vi "Keithley 2600 Series Current Sweep Script.vi"() -> ()   [LabVIEW 2020]
doc: "This example shows how to create, run a script and query the script output data."
uses:
  Keithley 2600 Series.lvlib
panel:
  out "Array":string[](array[string])
  out "error out":errorcluster
  out "Last Measured Voltage (V)":dbl
  out "Voltage Measurements (V)":string
  in  "Source Code":string="smua.reset()\nsmua.source.limitv = 1\nSweepILinMeasureV(smua, 0.01, 0.1, 0.2, 10)\nprintbuffer(1, 10, smua.nvbuffer1)\nprint(smua.nvbuffer1.readings[10])\n"
  in  "Script Variable (myScript)":string="myScript"
  in  "VISA resource name":refnum<visa-resource-name>
  # "(c) 2020 National Instruments.  ALL RIGHTS RESERVED."
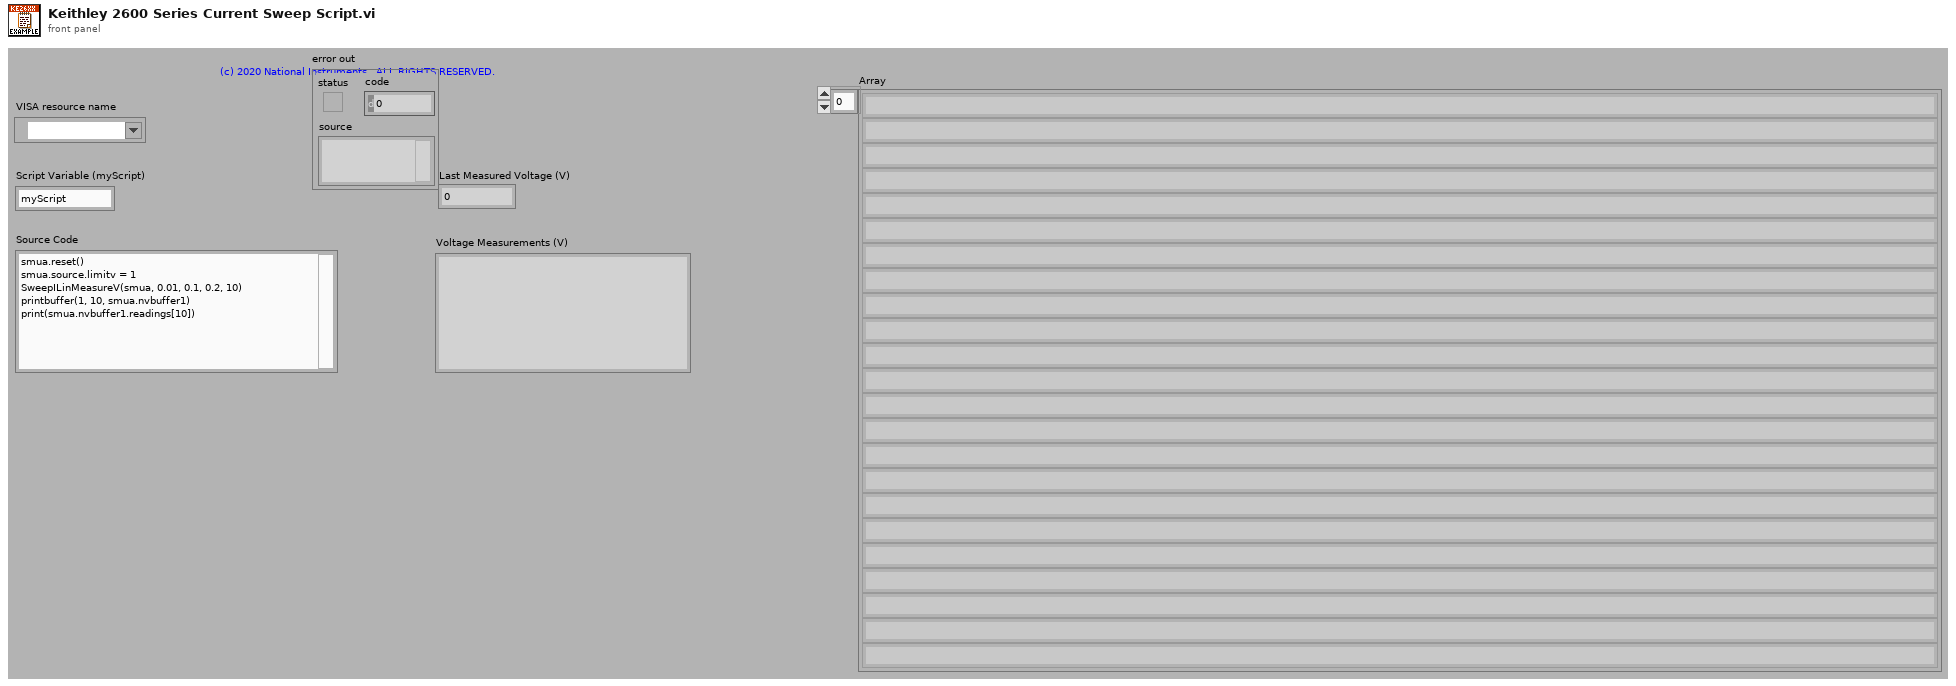
[diagram p1: front panel]
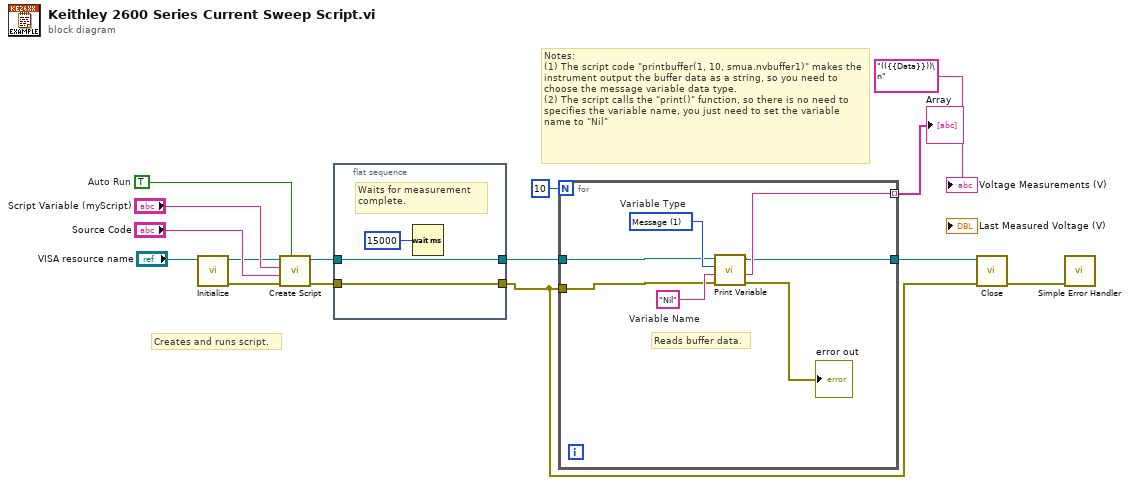
[diagram p0: block diagram]
diagram:
  w12 = TRUE  # Auto Run
  # "Notes: \n(1) The script code \"printbuffer(1, 10, smua.nvbuffer1)\" makes the instrument output the buffer data as a string, so you need to choose the message variable data type.\n(2) The script calls the \"print()\" function, so there is no need to specifies the variable name, you just need to set the variable name to \"Nil\""
  # "Creates and runs script."
  n1 = call "Initialize.vi"("VISA resource name"="VISA resource name") -> ("error out"=w7:errorcluster, "VISA resource name out"=w8:refnum<visa-resource-name>)  [unwired: 9 in]
  n2 = call <instrlib>:"Create Script.vi"("Auto Run (F: Disable)"=w12, "error in (no error)"=w7, "Source Code"="Source Code", "Script Variable"="Script Variable (myScript)", "VISA resource name"=w8) -> ("error out"=w10:errorcluster, "VISA resource name out"=w11:refnum<visa-resource-name>)  [unwired: 5 in]
  n3 = flat-sequence {
    tunnel: w11 -> [w16]
    tunnel: w10 -> [w17]
    tunnel: [w17] -> w6
    tunnel: [w16] -> w2
    frame #0 {
      # "Waits for measurement complete."
      n4 = Wait (ms)(milliseconds to wait=15000) -> ()  [unwired: 1 out]
    }
  }
  n5 = for {
    N: 10 -> [_]
    tunnel: w2 -> [w23]
    tunnel: w6 -> [w22]
    tunnel: [w21] -> w5 mode=indexing
    tunnel: [w19] -> w1
    w25 = 1 items=["Number", "Message"]  # Variable Type
    w24 = "Nil"  # Variable Name
    # "Reads buffer data."
    n6 = call <instrlib>:"Print Variable.vi"("error in (no error)"=w22, "Variable Name"=w24, "Variable Type (0: Number)"=w25, "VISA resource name"=w23) -> ("error out"=→"error out":errorcluster, "Message"=w21:string, "VISA resource name out"=w19:refnum<visa-resource-name>)  [unwired: 4 in, 1 out]
  }
  "Array" <- w5
  n7 = call "Close.vi"("error in (no error)"=w6, "VISA resource name"=w1) -> ("error out"=w13:errorcluster)  [unwired: 9 in]
  n8 = call <vilib>:"Simple Error Handler.vi"("error in (no error)"=w13) -> ()  [unwired: 4 in, 5 out]
  "Voltage Measurements (V)" <- "(({{Data}}))\n" ("Voltage Measurements (V)")
